vi "Test Resume.vi"(11 "Error in":errorcluster) -> (15 "Error out":errorcluster)   [LabVIEW 2020, in "StopWatchTests.lvlib"]
doc: "This VI is used for validating resume button in stopwatch"
uses:
  StopWatchTests.lvlib
  <vilib>/SLL Drona/APIs/Stimulus/ControlValue/SetValueAuto.vi
  <vilib>/SLL Drona/APIs/Get/GetControlValue/GetControlValueByPathString.vi
  <vilib>/SLL Drona/APIs/Assert/AssertControlValue/Equal.vi
  <vilib>/SLL Drona/APIs/Assert/AssertControlValue/GreaterOrEqual.vi
  <vilib>/SLL Drona/APIs/Stimulus/VI/CloseVI.vi
  <vilib>/addons/_JKI Toolkits/Caraya/classes/Test/Test.lvclass
  <vilib>/SLL Drona/Drona.lvlib
  <vilib>/SLL Drona/APIs/Stimulus/ControlValue/ControlValue.lvlib
  <vilib>/SLL Drona/APIs/Assert/AssertControlValue/AssertControlValue.lvlib
  <vilib>/SLL Drona/APIs/Get/GetControlValue/GetControlValue.lvlib
  <vilib>/SLL Drona/APIs/Stimulus/VI/VI.lvlib
panel:
  # "RESUME TEST"
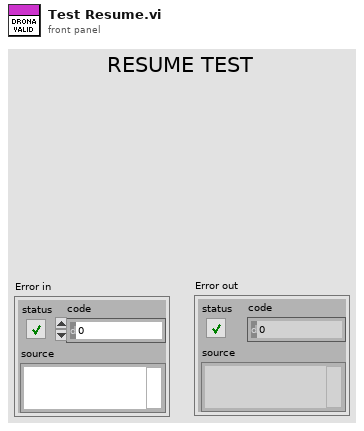
[diagram p1: front panel]
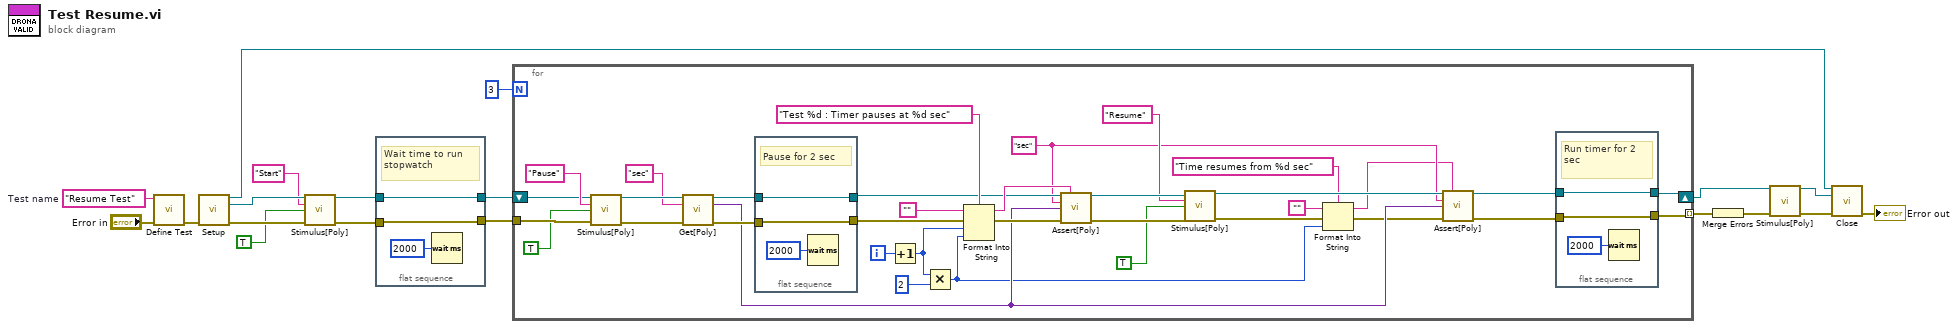
[diagram p0: block diagram]
diagram:
  w18 = "Resume Test"  # Test name
  n1 = call <vilib>:"Define Test.vi"("error in (no error)"="Error in", "Label (VI Title)"=w18) -> ("error out"=w17:errorcluster)  [unwired: 9 in]
  n2 = call <vilib>:"Setup.vi"("error in"=w17) -> ("Application Ref"=w15:refnum<vi>, "VI Reference Out"=w10:refnum<vi>, "error out"=w11:errorcluster)  [unwired: 12 in]
  n3 = call-poly <vilib>:"Stimulus[Poly].vi"("VI Reference In"=w10, "Control Path"="Start", "Value (Signaling)"=TRUE, "error in"=w11) -> ("VI Reference Out"=w6:refnum<vi>, "error out"=w7:errorcluster)  [unwired: 10 in]
  n4 = flat-sequence {
    tunnel: w7 -> [w21]
    tunnel: [w21] -> w5
    tunnel: w6 -> [w20]
    tunnel: [w20] -> w1
    frame #0 {
      # "Wait time to run  stopwatch"
      n5 = Wait (ms)(milliseconds to wait=u32 2000) -> ()  [unwired: 1 out]
    }
  }
  n6 = for {
    N: 3 -> [_]
    tunnel: w5 -> [w57]
    shift-right: [w41] -> w2
    shift-left: w1 -> [w39]
    tunnel: [w40] -> w4 mode=indexing
    i -> [w50]
    w31 = "sec" ("Control Path")
    n7 = call-poly <vilib>:"Stimulus[Poly].vi"("VI Reference In"=w39, "Control Path"="Pause", "Value (Signaling)"=TRUE, "error in"=w57) -> ("VI Reference Out"=w35:refnum<vi>, "error out"=w38:errorcluster)  [unwired: 10 in]
    n8 = call-poly <vilib>:"Get[Poly].vi"("VI Reference In"=w35, "Control Path"="sec", "error in"=w38) -> ("VI Reference Out"=w36:refnum<vi>, "Value"=w30:variant, "error out"=w37:errorcluster)  [unwired: 10 in]
    n9 = flat-sequence {
      tunnel: w37 -> [w62]
      tunnel: [w62] -> w54
      tunnel: w36 -> [w61]
      tunnel: [w61] -> w48
      frame #0 {
        # "Pause for 2 sec"
        n10 = Wait (ms)(milliseconds to wait=u32 2000) -> ()  [unwired: 1 out]
      }
    }
    n11 = Increment(x=w50) -> (x+1=w47:i32)
    n12 = Multiply(x=w47, y=2) -> (x*y=w24:i32)
    n13 = Format Into String(format string="Test %d : Timer pauses at %d sec", initial string="", error in=w54, w47, w24) -> (resulting string=w49:string, error out=w53:errorcluster)
    n14 = call-poly <vilib>:"Assert[Poly].vi"("VI Reference In"=w48, "Test Label"=w49, "Control Path"=w31, "Control Value"=w30, "Error In"=w53) -> ("VI Reference Out"=w45:refnum<vi>, "Error Out"=w44:errorcluster)  [unwired: 9 in]
    n15 = call-poly <vilib>:"Stimulus[Poly].vi"("VI Reference In"=w45, "Control Path"="Resume", "Value (Signaling)"=TRUE, "error in"=w44) -> ("VI Reference Out"=w32:refnum<vi>, "error out"=w33:errorcluster)  [unwired: 10 in]
    n16 = Format Into String(format string="Time resumes from %d sec" ("Test Label"), initial string="", error in=w33, w24) -> (resulting string=w23:string, error out=w27:errorcluster)
    n17 = call-poly <vilib>:"Assert[Poly].vi"("VI Reference In"=w32, "Test Label"=w23, "Control Path"=w31, "Control Value"=w30, "Error In"=w27) -> ("VI Reference Out"=w29:refnum<vi>, "Error Out"=w28:errorcluster)  [unwired: 9 in]
    n18 = flat-sequence {
      tunnel: w28 -> [w59]
      tunnel: [w59] -> w40
      tunnel: w29 -> [w58]
      tunnel: [w58] -> w41
      frame #0 {
        # "Run timer for 2 sec"
        n19 = Wait (ms)(milliseconds to wait=u32 2000) -> ()  [unwired: 1 out]
      }
    }
  }
  n20 = Merge Errors(w4) -> (w3:errorcluster)
  n21 = call-poly <vilib>:"Stimulus[Poly].vi"("VI Reference In"=w2, "error in"=w3) -> ("VI Reference Out"=w14:refnum<vi>, "error out"=w13:errorcluster)  [unwired: 12 in]
  n22 = call <vilib>:"Close.vi"("Application Ref"=w15, "VI Reference"=w14, "error in"=w13) -> ("error out"=→"Error out":errorcluster)  [unwired: 12 in]
